vi "IECMemory.LoadData.vi"(0 "i ref in":refnum<vi>, 2 "MemoryTimingArray":i32[][](array[numeric])=[[-1, 0], [-1, 0], [-1, 0], [-1, 0], [-1, 0], [-1, 0], [-1, 0], [-1, 0], [-1, 0], [-1, 0], [-1, 0], [-1, 0], [-1, 0]], 3 "ms timeout (100)":i32=100, 5 "error in (no error)":errorcluster) -> (14 "i ref out":refnum<vi>, 17 "timed out":bool, 19 "error out":errorcluster)   [LabVIEW 2014, in "IECMemory.lvlib"]
uses:
  IECMemory.lvlib
  CS_Core/CSSystem/CoreDefs/CoreDefs.error_type.ctl
  CS_Core/CSSystem/CoreLib/CoreLib.lvlib
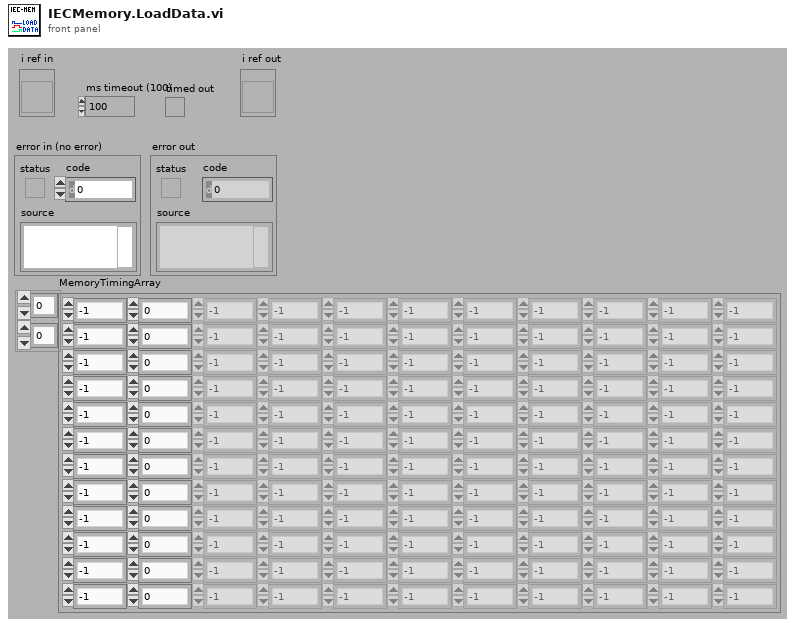
[diagram p1: front panel]
types:
  T1 = typedef "CoreDefs.error_type.ctl" = enum16{"no error", "can't load process", "can't unload process", "process does not exist", "can't install process", "can't remove process", "unknown function", "time out", "can't execute function", "duplicate queue name", "super not found", "caller queue invalid", "can't ping process", "unknown error", "VISA Error", "VISA timeout", "GPIB timeout", "GPIB error", "communication error", "data type mismatch", "can't read data from OPC server", "can't write data to OPC server", "OET error", "function not implemented", "process already exists", "invalid Shared Variable name", "error writing Shared Variable", "error reading Shared Variable", "invalid client name", "corrupt database", "unknown class", "call not authorized", "parameter out of range", "OET timeout: can't get data to modify", "invalid queue name", "requested operation incompatible with current state", "event undefined", "event disabled", "state undefined", "caller is not a friend", "EventBuilder: bad eventID", "EventBuilder: no DAQ devices", "a thread must not stop itself", "UNUSED ELEMENT4", "DiscArchiver: eventData incomplete", "DiscArchiver: eventData does not belong to run", "DiscArchiver: can't open file", "DiscArchiver: can't write to file", "DiscArchiver: available disc space low", "can't acquire semaphore", "error reading data from database", "notifier object is not existing", "can't register process", "can't unregister process", "illegal event type", "object disabled", "object already exists", "can't change state", "Instrument not found", "no connection to remote node", "invalid reference", "N/A", "UNUSED ELEMENT 1", "element not found", "illegal TCP/IP connection detected", "object does not exist", "invalid access ID", "unknown CS system", "invalid privilige", "unsupported data type", "unsupported server type", "IO server already exists", "Shared Variable already exists"}
  T2 = typedef "IECMemory.lvlib/IECMemory.i attribute.ctl" = cluster{"EndAddress":u32, "MemoryStatusBits":T3, "IEC Finished":bool, "Call Process":string, "Call Event":string}
  T3 = typedef "IECMemoryDriver.lvlib/Memory_Status.ctl" = bool[]
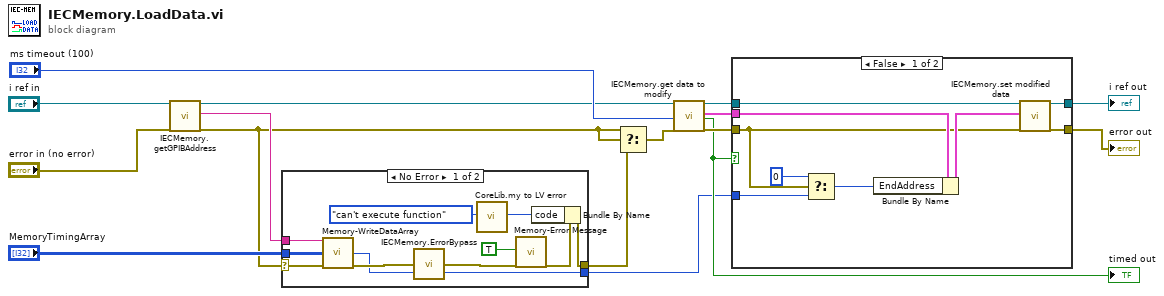
[diagram p0: block diagram]
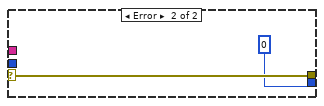
[diagram p2: hidden frame]
diagram:
  n1 = call "IECMemory.getGPIBAddress.vi"("i ref in"="i ref in", "error in (no error)"="error in (no error)") -> ("i ref out"=w10:refnum<vi>, "GPIBAddress"=w6:string, "error out"=w2:errorcluster)  [unwired: 14 in, 1 out]
  n2 = case shown="No Error" w2 {
    selector: w2 -> [w22 w29]
    tunnel: [w24 w29] -> w1
    tunnel: [w18 u32 0] -> w4
    tunnel: w6 -> [w20 _]
    tunnel: "MemoryTimingArray" -> [w19 _]
    frame No Error {
      n3 = call "Memory-WriteDataArray.vi"("AddressStringIN"=w20, "MemoryTimingArray"=w19, "error in (no error)"=w22) -> ("EndAddress"=w18:i16, "error out"=w21:errorcluster)  [unwired: 11 in]
      n4 = call "IECMemory.ErrorBypass.vi"("error in (no error)"=w21) -> ("error out"=w17:errorcluster)  [unwired: 14 in]
      n5 = call "CoreLib.my to LV error.vi"("ErrorTypes"=CoreDefs.error_type."can't execute function") -> ("LV error code"=w23:i32)  [unwired: 17 in, 1 out]
      n6 = call "Memory-Error Message.vi"("add message to source"=TRUE, "error in (no error)"=w17) -> ("error out"=w25:errorcluster)  [unwired: 14 in, 3 out]
      n7 = Bundle By Name(cluster=w25, "code"=w23) -> (w24:errorcluster)
    }
    frame Error {
    }
  }
  n8 = Select(t=w2, s=w2, f=w1) -> (s? t:f=w3:errorcluster)
  n9 = call "IECMemory.get data to modify.vi"("i ref in"=w10, "ms timeout (10000)"="ms timeout (100)", "error in (no error)"=w3) -> ("i ref out"=w14:refnum<vi>, "i attribute"=w12:T2, "timed out"=w9:bool, "error out"=w13:errorcluster)  [unwired: 13 in]
  "timed out" <- w9
  n10 = case shown="False" w9 {
    tunnel: w14 -> [w34 w40]
    tunnel: [w36 w40] -> w8
    tunnel: [w35 w39] -> w7
    tunnel: w13 -> [w32 w39]
    tunnel: w12 -> [w38 _]
    tunnel: w4 -> [w30 _]
    frame False {
      n11 = Select(t=u32 0, s=w32, f=w30) -> (s? t:f=w37:u32)
      n12 = Bundle By Name(cluster=w38, "EndAddress"=w37) -> (w33:T2)
      n13 = call "IECMemory.set modified data.vi"("i ref in"=w34, "i attribute"=w33, "error in (no error)"=w32) -> ("i ref out"=w36:refnum<vi>, "error out"=w35:errorcluster)  [unwired: 15 in]
    }
    frame True {
    }
  }
  "error out" <- w7
  "i ref out" <- w8
